vi "DMM_Mixed Meas Initialize.vi"(0 "DMM Resource Name":refnum<k15>, 2 "Powerline Frequency":T1=enum."50 Hz", 11 "error in":errorcluster) -> (4 "DMM Handle Out":refnum<k15>, 15 "error out":errorcluster)   [LabVIEW 2021, in "DMM_Mixed Measurement.lvlib"]
doc: "Creates a new NI-DMM driver session on the device specified in the DMM Resource Name control configured with the local powerline frequency. The device uses the powerline frequency value to select a timebase for setting the Aperture Time property in powerline cycles (PLCs). Change Powerline Frequency value to 60 Hz for North & South America."
uses:
  DMM_Mixed Measurement.lvlib
  <instrlib>/niDMM/nidmm.llb/niDMM Powerline Frequency.ctl
panel:
  # "Inputs"
  # "Outputs"
  # "Overview:\nThis VI interacts with the NI-DMM driver to initialize an NI DMM instrument and provide a corresponding instrument handle\n\nHardware Requirements: A PXI, PCIe, or USB DMM instrument\n\nSoftware Requirements: NI DMM 2022 Q3 or above\n\nInstructions:\nSelect your DMM instrument resource name in the drop down control\n\nNote: The \"DMM Handle Out\" indicator will be used by the Configure & Measure and Close API functions"
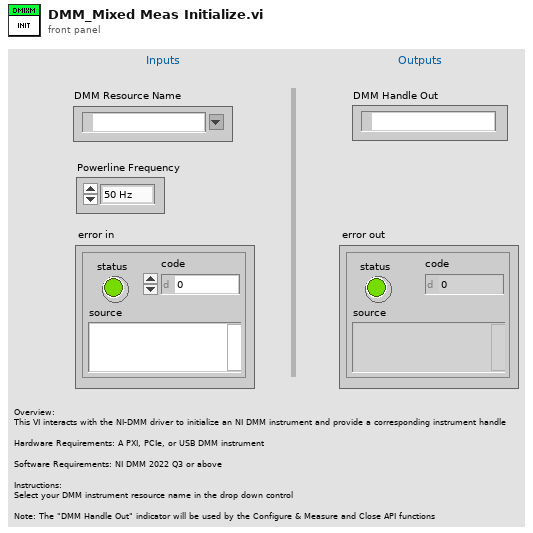
[diagram p1: front panel]
types:
  T1 = typedef "niDMM Powerline Frequency.ctl" = enum16{"60 Hz", "50 Hz"}
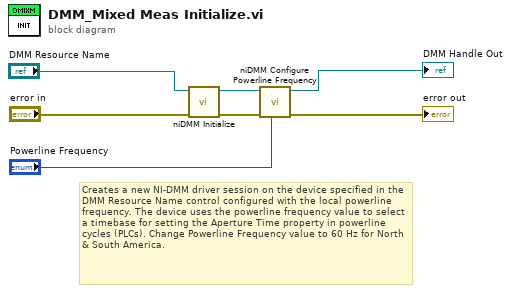
[diagram p0: block diagram]
diagram:
  # "Creates a new NI-DMM driver session on the device specified in the DMM Resource Name control configured with the local powerline frequency. The device uses the powerline frequency value to select a timebase for setting the Aperture Time property in powerline cycles (PLCs). Change Powerline Frequency value to 60 Hz for North & South America."
  n1 = call <instrlib>:"niDMM Initialize.vi"("error in (no error)"="error in", "Instrument Descriptor"="DMM Resource Name") -> ("error out"=w5:errorcluster, "instrument handle out"=w4:refnum<k15>)  [unwired: 8 in]
  n2 = call <instrlib>:"niDMM Configure Powerline Frequency.vi"("Powerline Frequency"="Powerline Frequency", "error in (no error)"=w5, "instrument handle"=w4) -> ("error out"=→"error out":errorcluster, "instrument handle out"=→"DMM Handle Out":refnum<k15>)  [unwired: 7 in]
